vi "read_bianry.vi"() -> ()   [LabVIEW 2021]
panel:
  out "data":i32[](array[numeric])
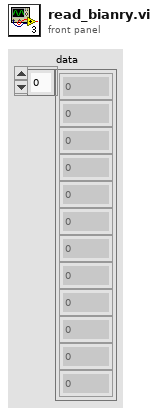
[diagram p1: front panel]
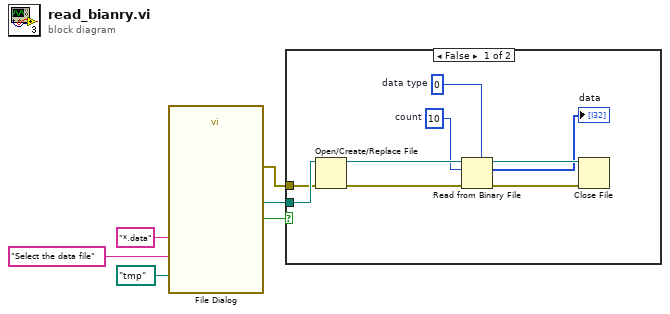
[diagram p0: block diagram]
diagram:
  n1 = call "File Dialog"("start path"=path "/tmp", "prompt"="Select the data file", "pattern (all files)"="*.data" ("pattern label")) -> ("selected path"=w5:path, "cancelled"=w1:bool, "error out"=w4:errorcluster)  [unwired: 9 in, 1 out]
  n2 = case shown="False" w1 {
    tunnel: w5 -> [w11 _]
    tunnel: w4 -> [w7 _]
    frame False {
      w10 = 0  # data type
      w9 = 10  # count
      n3 = Open/Create/Replace File(file path (use dialog)=w11, error in=w7) -> (refnum out=w12:refnum<file>, error out=w13:errorcluster)  [unwired: 4 in, 1 out]
      n4 = Read from Binary File(5:w10, 8:w13, 10:w9, 11:w12) -> (0:w15:errorcluster, 2:→"data":i32[], 3:w14:refnum<file>)  [unwired: 2 in, 1 out]
      n5 = Close File(refnum=w14, error in=w15) -> ()  [unwired: 2 out]
    }
    frame True {
    }
  }
